vi "arduino.vi"() -> ()   [LabVIEW 2020]
panel:
  out "read buffer":string
  in  "Boolean":bool
  in  "write buffer":string
  in  "stop":bool
  in  "VISA resource name":refnum<visa-resource-name>
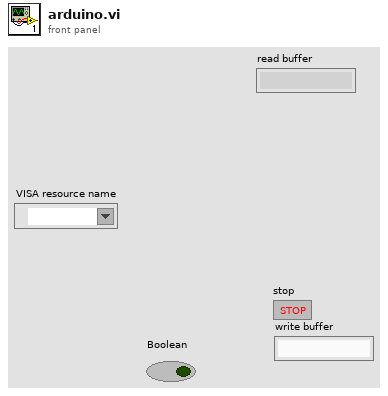
[diagram p1: front panel]
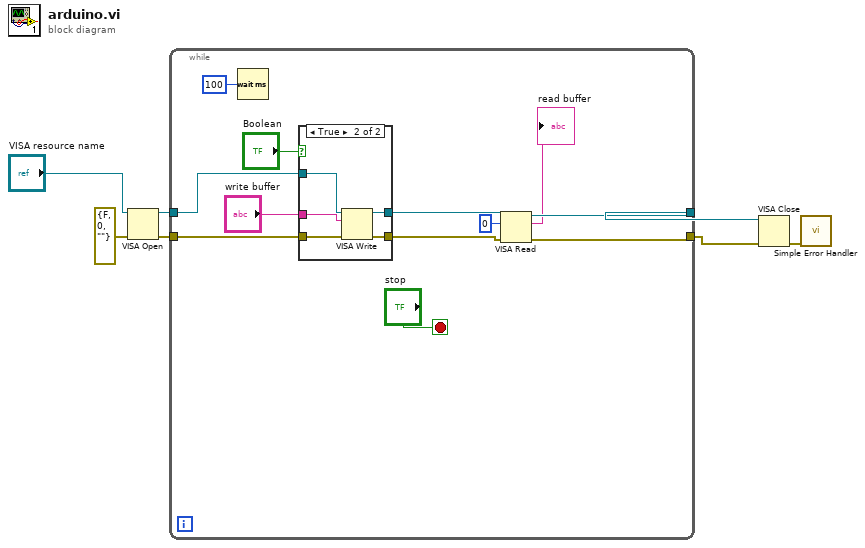
[diagram p0: block diagram]
diagram:
  n1 = VISA Open(error in (no error)=errorcluster {"status"=FALSE, "code"=0, "source"=""}, VISA resource name="VISA resource name") -> (VISA resource name=w6:refnum<visa-resource-name>, error out=w5:errorcluster)  [unwired: 3 in]
  n2 = while {
    tunnel: w6 -> [w18]
    tunnel: w5 -> [w17]
    tunnel: [w11] -> w4
    tunnel: [w10] -> w1
    stop <- "stop" stop-if-true
    n3 = Wait (ms)(milliseconds to wait=u32 100) -> ()  [unwired: 1 out]
    n4 = case shown="True" "Boolean" {
      tunnel: w18 -> [w20 w26]
      tunnel: w17 -> [w21 w25]
      tunnel: [w20 w24] -> w12
      tunnel: "write buffer" -> [_ w23]
      tunnel: [w21 w22] -> w13
      frame False {
      }
      frame True {
        n5 = VISA Write(VISA resource name=w26, write buffer=w23, error in (no error)=w25) -> (VISA resource name out=w24:refnum<visa-resource-name>, error out=w22:errorcluster)  [unwired: 1 out]
      }
    }
    n6 = VISA Read(VISA resource name=w12, byte count=u32 0, error in (no error)=w13) -> (VISA resource name out=w11:refnum<visa-resource-name>, read buffer=→"read buffer":string, error out=w10:errorcluster)  [unwired: 1 out]
  }
  n7 = VISA Close(VISA resource name=w4, error in (no error)=w1) -> (error out=w2:errorcluster)
  n8 = call <vilib>:"Simple Error Handler.vi"("error in (no error)"=w2) -> ()  [unwired: 4 in, 5 out]
